vi "NI 9476_TASK_DO.vi"(8 "error in":errorcluster, 11 "MODULE NAME":string="cDAQ_NICOTRAMod2") -> (0 "error out":errorcluster, 3 "task out":refnum<k21>)   [LabVIEW 2016]
uses:
  <vilib>/DAQmx/create/channels.llb/DAQmx Create Channel (DO-Digital Output).vi
  <resource>/objmgr/daqmx.rc
panel:
  out "Numeric":i32
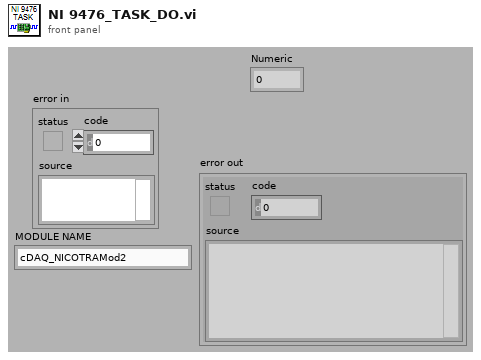
[diagram p1: front panel]
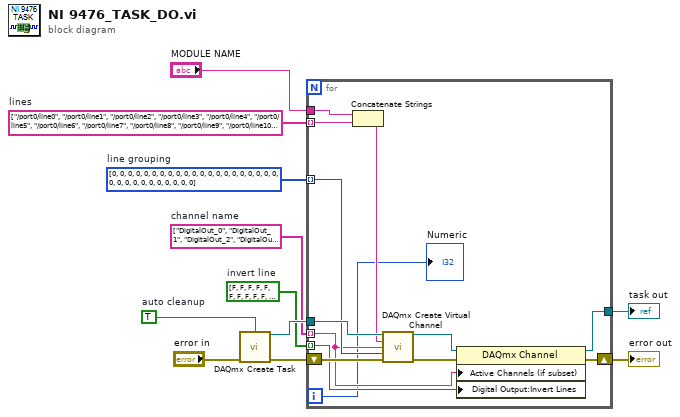
[diagram p0: block diagram]
diagram:
  w7 = bool[] [FALSE, FALSE, FALSE, FALSE, FALSE, FALSE, FALSE, FALSE, FALSE, FALSE, FALSE, FALSE, FALSE, FALSE, FALSE, FALSE, FALSE, FALSE, FALSE, FALSE, FALSE, FALSE, FALSE, FALSE, FALSE, FALSE, FALSE, FALSE, FALSE, FALSE, FALSE, FALSE]  # invert line
  w6 = i32[] [0, 0, 0, 0, 0, 0, 0, 0, 0, 0, 0, 0, 0, 0, 0, 0, 0, 0, 0, 0, 0, 0, 0, 0, 0, 0, 0, 0, 0, 0, 0, 0] items=["one channel for each line", "one channel for all lines"]  # line grouping
  w5 = string[] ["DigitalOut_0", "DigitalOut_1", "DigitalOut_2", "DigitalOut_3", "DigitalOut_4", "DigitalOut_5", "DigitalOut_6", "DigitalOut_7", "DigitalOut_8", "DigitalOut_9", "DigitalOut_10", "DigitalOut_11", "DigitalOut_12", "DigitalOut_13", "DigitalOut_14", "DigitalOut_15", "DigitalOut_16", "DigitalOut_17", "DigitalOut_18", "DigitalOut_19", "DigitalOut_20", "DigitalOut_21", "DigitalOut_22", "DigitalOut_23", "DigitalOut_24", "DigitalOut_25", "DigitalOut_26", "DigitalOut_27", "DigitalOut_28", "DigitalOut_29", "DigitalOut_30", "DigitalOut_31"]  # channel name
  w4 = string[] ["/port0/line0", "/port0/line1", "/port0/line2", "/port0/line3", "/port0/line4", "/port0/line5", "/port0/line6", "/port0/line7", "/port0/line8", "/port0/line9", "/port0/line10", "/port0/line11", "/port0/line12", "/port0/line13", "/port0/line14", "/port0/line15", "/port0/line16", "/port0/line17", "/port0/line18", "/port0/line19", "/port0/line20", "/port0/line21", "/port0/line22", "/port0/line23", "/port0/line24", "/port0/line25", "/port0/line26", "/port0/line27", "/port0/line28", "/port0/line29", "/port0/line30", "/port0/line31"]  # lines
  w9 = TRUE  # auto cleanup
  n1 = call <vilib>:"DAQmx Create Task.vi"("auto cleanup"=w9, "error in"="error in") -> ("task out"=w8:refnum<k21>, "error out"=w10:errorcluster)  [unwired: 12 in]
  n2 = for {
    tunnel: w8 -> [w24]
    tunnel: w7 -> [w19] mode=indexing
    tunnel: w6 -> [w22] mode=indexing
    tunnel: w5 -> [w18] mode=indexing
    tunnel: w4 -> [w15] mode=indexing
    tunnel: [w20] -> w3
    shift-right: [w16] -> w2
    shift-left: w10 -> [w23]
    tunnel: "MODULE NAME" -> [w14]
    i -> [w12]
    n3 = Concatenate Strings(w14, w15) -> (w13:string)
    n4 = call-poly <vilib>:"DAQmx Create Virtual Channel.vi"("task in"=w24, "lines"=w13, "name to assign"=w18, "line grouping"=w22, "error in"=w23) -> ("task out"=w21:refnum<k21>, "error out"=w17:errorcluster)  [unwired: 9 in]
    n5 = property class="DAQmx Channel"(reference=w21, error in=w17, "Active Channels (if subset)"=w18, "Digital Output:Invert Lines"=w19) -> (reference out=w20:refnum<k21>, error out=w16:errorcluster)
    "Numeric" <- w12
  }
  "error out" <- w2
  "task out" <- w3
